vi "dcimg_to_tif.vi"(8 "error in (no error)":errorcluster, 9 "Where to Store":path, 11 "DCIMG Path":path) -> (0 "Error Out":errorcluster, 3 "Index":i32)   [LabVIEW 2017]
panel:
  out "Total":i32
  # "This is an example of how to read the images\nwithin a DCIMG file and write them to TIFF files."
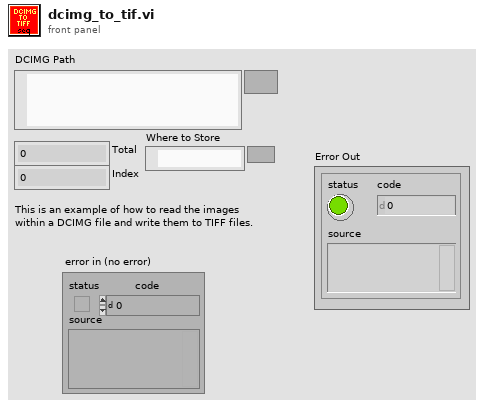
[diagram p1: front panel]
types:
  T1 = typedef "Image Type" = u32
  T2 = typedef "IMAQ Image.ctl" = refnum<image>
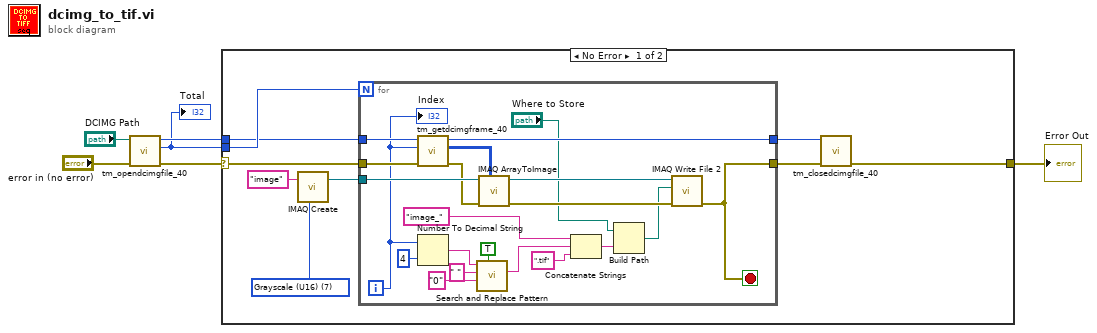
[diagram p0: block diagram]
diagram:
  n1 = call <userlib>:"tm_opendcimgfile_40.vi"("error in (no error)"="error in (no error)", "Path"="DCIMG Path") -> ("error out"=w6:errorcluster, "Total Frames"=w3:i32, "File Handle"=w5:u32)  [unwired: 7 in]
  "Total" <- w3
  n2 = case shown="No Error" w6 {
    selector: w6 -> [w12 w37]
    tunnel: w5 -> [w13 _]
    tunnel: [w15 w37] -> w2
    tunnel: w3 -> [w14 _]
    frame No Error {
      w10 = T1 7 items=["Grayscale (U8)", "Grayscale (I16)", "Grayscale (SGL)", "Complex (CSG)", "RGB (U32)", "HSL (U32)", "RGB (U64)", "Grayscale (U16)"] ("Image Type")
      n3 = call "IMAQ Create"("Image Name"="image", "Image Type"=w10) -> ("New Image"=w9:T2)  [unwired: 3 in, 1 out]
      n4 = for {
        N: w14 -> [_]
        tunnel: w13 -> [w36]
        tunnel: w12 -> [w35]
        tunnel: w9 -> [w34]
        tunnel: [w17] -> w7
        tunnel: [w30] -> w8
        i -> [w18]
        stop <- w17 stop-if-true
        n5 = call <userlib>:"tm_getdcimgframe_40.vi"("error in (no error)"=w35, "Frame Index"=w18, "File Handle in"=w36) -> ("error out"=w31:errorcluster, "Data"=w19:u16[][], "File Handle out"=w30:u32)  [unwired: 5 in, 1 out]
        n6 = Number To Decimal String(number=w18, width (-)=i16 4) -> (decimal integer string=w27:string)
        n7 = call <vilib>:"Search and Replace Pattern.vi"("string"=w27, "regular expression (\"\")"=" " ("regular expression (\"\")"), "replace string (\"\")"="0" ("replace string (\"\")"), "replace all? (F)"=TRUE) -> ("result string"=w23:string)  [unwired: 1 in, 1 out]
        n8 = call "IMAQ ArrayToImage"("Image Pixels (U16)"=w19, "error in (no error)"=w31, "Image"=w34) -> ("error out"=w33:errorcluster, "Image Out"=w32:T2)  [unwired: 7 in]
        n9 = Concatenate Strings("image_", w23, ".tif" ("regular expression (\"\")")) -> (w22:string)
        n10 = Build Path(base path="Where to Store", name or relative path=w22) -> (appended path=w21:path)
        n11 = call-poly "IMAQ Write File 2"("error in (no error)"=w33, "File Path"=w21, "Image"=w32) -> ("error out"=w17:errorcluster)  [unwired: 7 in, 1 out]
        "Index" <- w18
      }
      n12 = call <userlib>:"tm_closedcimgfile_40.vi"("error in (no error)"=w7, "File Handle"=w8) -> ("error out"=w15:errorcluster)  [unwired: 9 in]
    }
    frame Error {
    }
  }
  "Error Out" <- w2
